vi "Read FIB Log Files.vi"(9 "Log file type":u8(ring) items=["HV Data", "Reheat"], 11 "Log file path":path=path "C:/Program Files (x86)/FEI Company/BDS/LogHVData.log") -> (1 "Reheat Output":T1 {"Initial suppressor (V)" format="%.1f"; "Initial emission (uA)" format="%.3f"; "V/I Slope" format="%.2f"}, 3 "HV Data Output":T2 {"Tip Lifetime (hr)" format="%.2f"; "Lens2I (uA)" format="%.3f"; "Lens2 (V)" format="%.1f"; "Lens1I (uA)" format="%.3f"; "Lens1 (V)" format="%.1f"; "SuppI (uA)" format="%.3f"; "Suppressor (V)" format="%.1f"; "Emission (uA)" format="%.3f"; "Extractor (V)" format="%.1f"; "AccI (uA)" format="%.3f"; "Acclerator (V)" format="%.1f"; "Filament (A)" format="%.2f"})   [LabVIEW 2018]
uses:
  <vilib>/regexp/Match Regular Expression.xnode
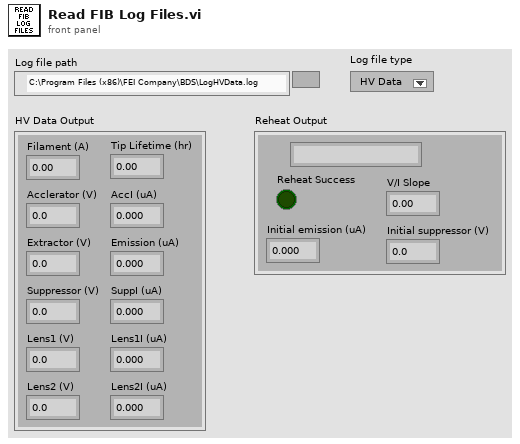
[diagram p1: front panel]
types:
  T1 = cluster{"Reheat finish time":string, "Reheat Success":bool, "Initial emission (uA)":sgl, "Initial suppressor (V)":sgl, "V/I Slope":sgl}
  T2 = cluster{"Filament (A)":sgl, "Acclerator (V)":sgl, "AccI (uA)":sgl, "Extractor (V)":sgl, "Emission (uA)":sgl, "Suppressor (V)":sgl, "SuppI (uA)":sgl, "Lens1 (V)":sgl, "Lens1I (uA)":sgl, "Lens2 (V)":sgl, "Lens2I (uA)":sgl, "Tip Lifetime (hr)":sgl}
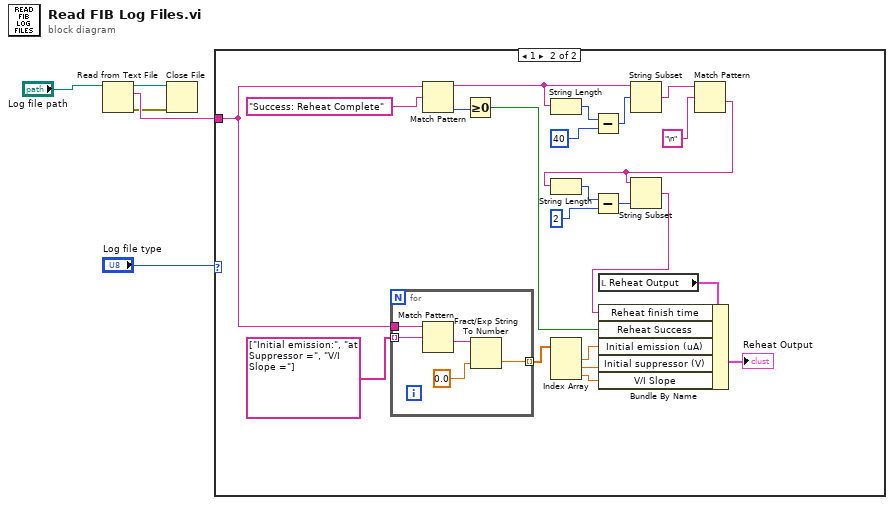
[diagram p0: block diagram]
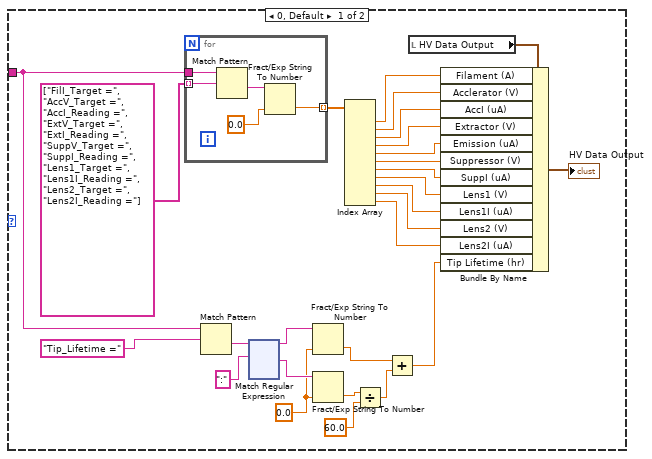
[diagram p2: hidden frame]
diagram:
  n1 = Read from Text File(file (use dialog)="Log file path") -> (refnum out=w2:refnum<file>, text=w4:string, error out=w3:errorcluster)  [unwired: 3 in, 1 out]
  n2 = Close File(refnum=w2, error in=w3) -> ()  [unwired: 2 out]
  n3 = case shown="1" "Log file type" {
    tunnel: w4 -> [w8 w161]
    frame 0, Default {
      w6 = sgl 0.0 ("default (0 DBL)")
      n4 = for {
        tunnel: string[] ["FilI_Target =", "AccV_Target =", "AccI_Reading =", "ExtV_Target =", "ExtI_Reading =", "SuppV_Target =", "SuppI_Reading =", "Lens1_Target =", "Lens1I_Reading =", "Lens2_Target =", "Lens2I_Reading ="] -> [w36] mode=indexing
        tunnel: w8 -> [w37]
        tunnel: [w33] -> w22 mode=indexing
        n5 = Match Pattern(string=w37, regular expression=w36) -> (after substring=w34:string)  [unwired: 1 in, 3 out]
        n6 = Fract/Exp String To Number(string=w34, default (0 dbl)=sgl 0.0 ("default (0 DBL)")) -> (number=w33:sgl)  [unwired: 3 out]
      }
      n7 = Match Pattern(string=w8, regular expression="Tip_Lifetime =") -> (after substring=w27:string)  [unwired: 1 in, 3 out]
      n8 = xnode "Match Regular Expression"("input string"=w27, "regular expression"=":") -> ("before match"=w26:string, "after match"=w31:string)  [unwired: 4 in, 3 out]
      n9 = Fract/Exp String To Number(string=w26, default (0 dbl)=w6) -> (number=w24:sgl)  [unwired: 3 out]
      n10 = Fract/Exp String To Number(string=w31, default (0 dbl)=w6) -> (number=w29:sgl)  [unwired: 3 out]
      n11 = Index Array(array=w22) -> (element #1=w20:sgl, element #2=w19:sgl, element #3=w18:sgl, element #4=w17:sgl, element #5=w16:sgl, element #6=w15:sgl, element #7=w14:sgl, element #8=w13:sgl, element #9=w12:sgl, element #10=w11:sgl, element #11=w10:sgl)  [unwired: 11 in]
      n12 = Divide(x=w29, y=sgl 60.0) -> (x/y=w25:sgl)
      n13 = Add(x=w24, y=w25) -> (x+y=w7:sgl)
      n14 = local read "HV Data Output"() -> (w21:T2)
      n15 = Bundle By Name(cluster=w21, "Filament (A)"=w20, "Acclerator (V)"=w19, "AccI (uA)"=w18, "Extractor (V)"=w17, "Emission (uA)"=w16, "Suppressor (V)"=w15, "SuppI (uA)"=w14, "Lens1 (V)"=w13, "Lens1I (uA)"=w12, "Lens2 (V)"=w11, "Lens2I (uA)"=w10, "Tip Lifetime (hr)"=w7) -> (→"HV Data Output":T2)
    }
    frame 1 {
      n16 = for {
        tunnel: string[] ["Initial emission:", "at Suppressor =", "V/I Slope ="] -> [w174] mode=indexing
        tunnel: w161 -> [w175]
        tunnel: [w171] -> w169 mode=indexing
        n17 = Match Pattern(string=w175, regular expression=w174) -> (after substring=w172:string)  [unwired: 1 in, 3 out]
        n18 = Fract/Exp String To Number(string=w172, default (0 dbl)=sgl 0.0 ("default (0 DBL)")) -> (number=w171:sgl)  [unwired: 3 out]
      }
      n19 = Match Pattern(string=w161, regular expression="Success: Reheat Complete") -> (before substring=w159:string, offset past match=w168:i32)  [unwired: 1 in, 2 out]
      n20 = Greater Or Equal To 0?(x=w168) -> (x >= 0?=w166:bool)
      n21 = String Length(string=w159) -> (length=w158:i32)
      n22 = Index Array(array=w169) -> (element #1=w165:sgl, element #2=w164:sgl, element #3=w163:sgl)  [unwired: 3 in]
      n23 = Subtract(x=w158, y=40) -> (x-y=w156:i32)
      n24 = local read "Reheat Output"() -> (w167:T1)
      n25 = String Subset(string=w159, offset (0)=w156) -> (substring=w155:string)  [unwired: 1 in]
      n26 = Match Pattern(string=w155, regular expression="\n") -> (after substring=w150:string)  [unwired: 1 in, 3 out]
      n27 = String Length(string=w150) -> (length=w153:i32)
      n28 = Subtract(x=w153, y=2) -> (x-y=w151:i32)
      n29 = String Subset(string=w150, length (rest)=w151) -> (substring=w149:string)  [unwired: 1 in]
      n30 = Bundle By Name(cluster=w167, "Reheat finish time"=w149, "Reheat Success"=w166, "Initial emission (uA)"=w165, "Initial suppressor (V)"=w164, "V/I Slope"=w163) -> (→"Reheat Output":T1)
    }
  }
